vi "Map_Get_Cell_Cost.vi"(8 "error in (no error)":errorcluster, 9 "Y_map":i32, 10 "X_map":i32, 11 "Map_in":dbl[][](array[numeric])) -> (0 "error out":errorcluster, 2 "cell cost":dbl, 3 "Map_out":dbl[][](array[numeric]))   [LabVIEW 2017]
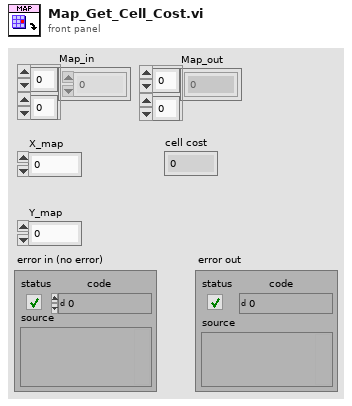
[diagram p1: front panel]
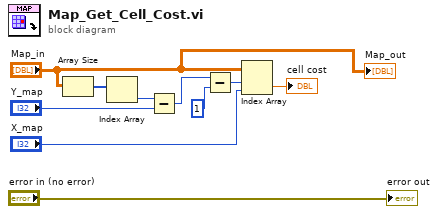
[diagram p0: block diagram]
diagram:
  n1 = Array Size(array="Map_in") -> (size(s)=w3:i32[])
  n2 = Index Array(array=w3) -> (element=w4:i32)  [unwired: 1 in]
  n3 = Subtract(x=w4, y="Y_map") -> (x-y=w6:i32)
  n4 = Subtract(x=w6, y=1) -> (x-y=w9:i32)
  n5 = Index Array(array="Map_in", index (row)=w9, index (col)="X_map") -> (element=→"cell cost":dbl)
  "Map_out" <- "Map_in"
  "error out" <- "error in (no error)"
